vi "AuMT8852B Wait for Operation to Complete.vi"(7 "Timeout (10000 ms)":i32=10000, 8 "error in (no error)":errorcluster, 11 "VISA session":refnum<visa-resource-name>) -> (0 "error out":errorcluster, 2 "error code":i32, 3 "VISA session out":refnum<visa-resource-name>)   [LabVIEW 2017]
doc: "Anritsu MT8852B Bluetooth Tester\n\nReturns when the instrument has completed the current operation."
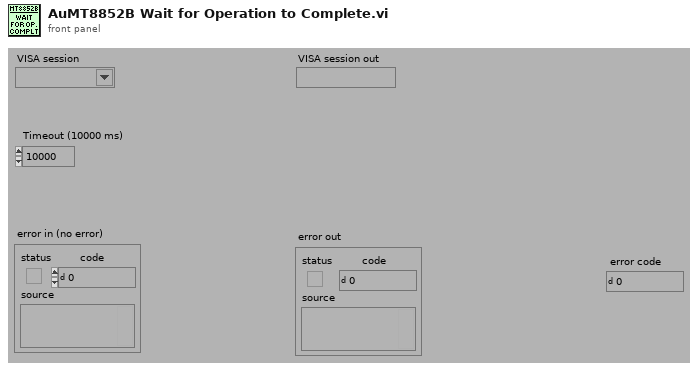
[diagram p1: front panel]
types:
  T1 = enum16{"Simulate", "Range check", "Cache", "Query instrument status"}
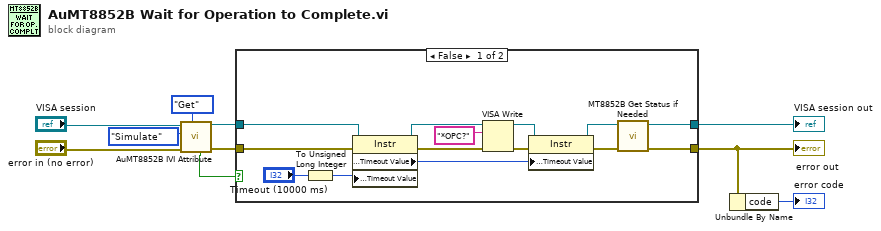
[diagram p0: block diagram]
diagram:
  n1 = call <instrlib>:"AuMT8852B IVI Attribute.vi"("Set/Get (Set)"=enum16{"Set", "Get"}."Get", "error in (no error)"="error in (no error)", "Flag (Simulate)"=T1."Simulate", "VISA session"="VISA session") -> ("error out"=w6:errorcluster, "VISA session out"=w7:refnum<visa-resource-name>, "Value out"=w3:bool)  [unwired: 5 in]
  n2 = case shown="False" w3 {
    tunnel: [w24 w25] -> w10
    tunnel: [w23 w26] -> w1
    tunnel: w7 -> [w21 w25]
    tunnel: w6 -> [w20 w26]
    frame False {
      n3 = To Unsigned Long Integer(number="Timeout (10000 ms)") -> (unsigned 32bit integer=w11:u32)
      n4 = property class="Instr"(reference=w21, error in=w20, "General Settings:Timeout Value"=w11) -> (reference out=w18:refnum<visa-resource-name>, error out=w17:errorcluster, "General Settings:Timeout Value"=w12:u32)
      n5 = VISA Write(VISA resource name=w18, write buffer="*OPC?" ("write buffer (\"\")"), error in (no error)=w17) -> (VISA resource name out=w15:refnum<visa-resource-name>, error out=w16:errorcluster)  [unwired: 1 out]
      n6 = property class="Instr"(reference=w15, error in=w16, "General Settings:Timeout Value"=w12) -> (reference out=w14:refnum<visa-resource-name>, error out=w13:errorcluster)
      n7 = call <instrlib>:"MT8852B Get Status if Needed.vi"("error in (no error)"=w13, "VISA session"=w14) -> ("error out"=w23:errorcluster, "VISA session out"=w24:refnum<visa-resource-name>)  [unwired: 8 in]
    }
    frame True {
    }
  }
  "VISA session out" <- w10
  "error out" <- w1
  n8 = Unbundle By Name(w1) -> ("code"=→"error code":i32)
